vi "girpcutil_GetMethodParams.vi"(6 "timeoutMs":u32=5000, 8 "Fehler (Eingang, kein Fehler)":errorcluster, 10 "methodName":string, 11 "girpcutil_params":T1) -> (0 "Fehler (Ausgang)":errorcluster, 2 "param handle out":i32)   [LabVIEW 2016]
uses:
  girpcutil_params.ctl
panel:
  out "errMsg":u8[](array[numeric])
  out "errMsgLen":i32
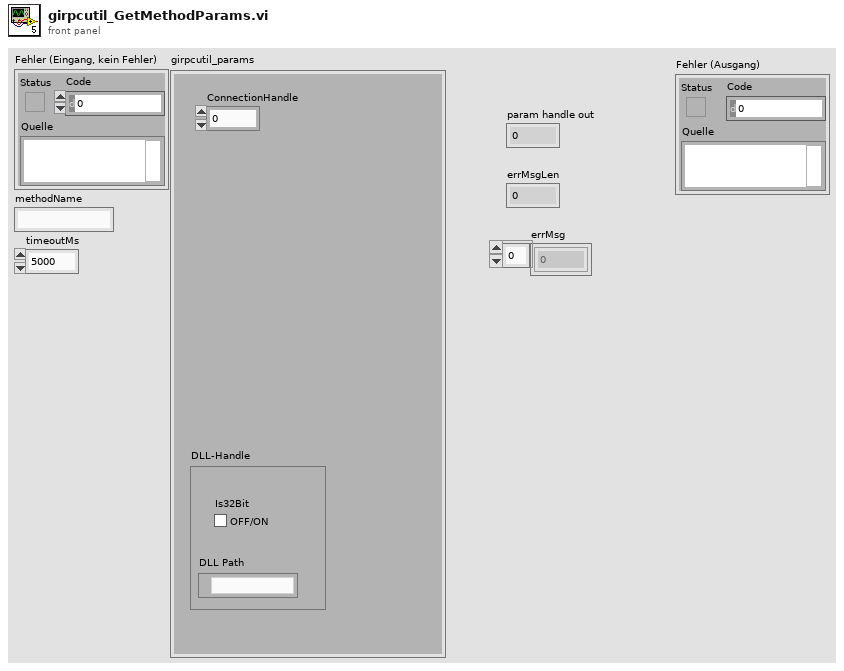
[diagram p1: front panel]
types:
  T1 = typedef "girpcutil_params.ctl" = cluster{"ConnectionHandle":i32, "DLL-Handle":cluster{"DLL Path":path, "Is32Bit":bool}}
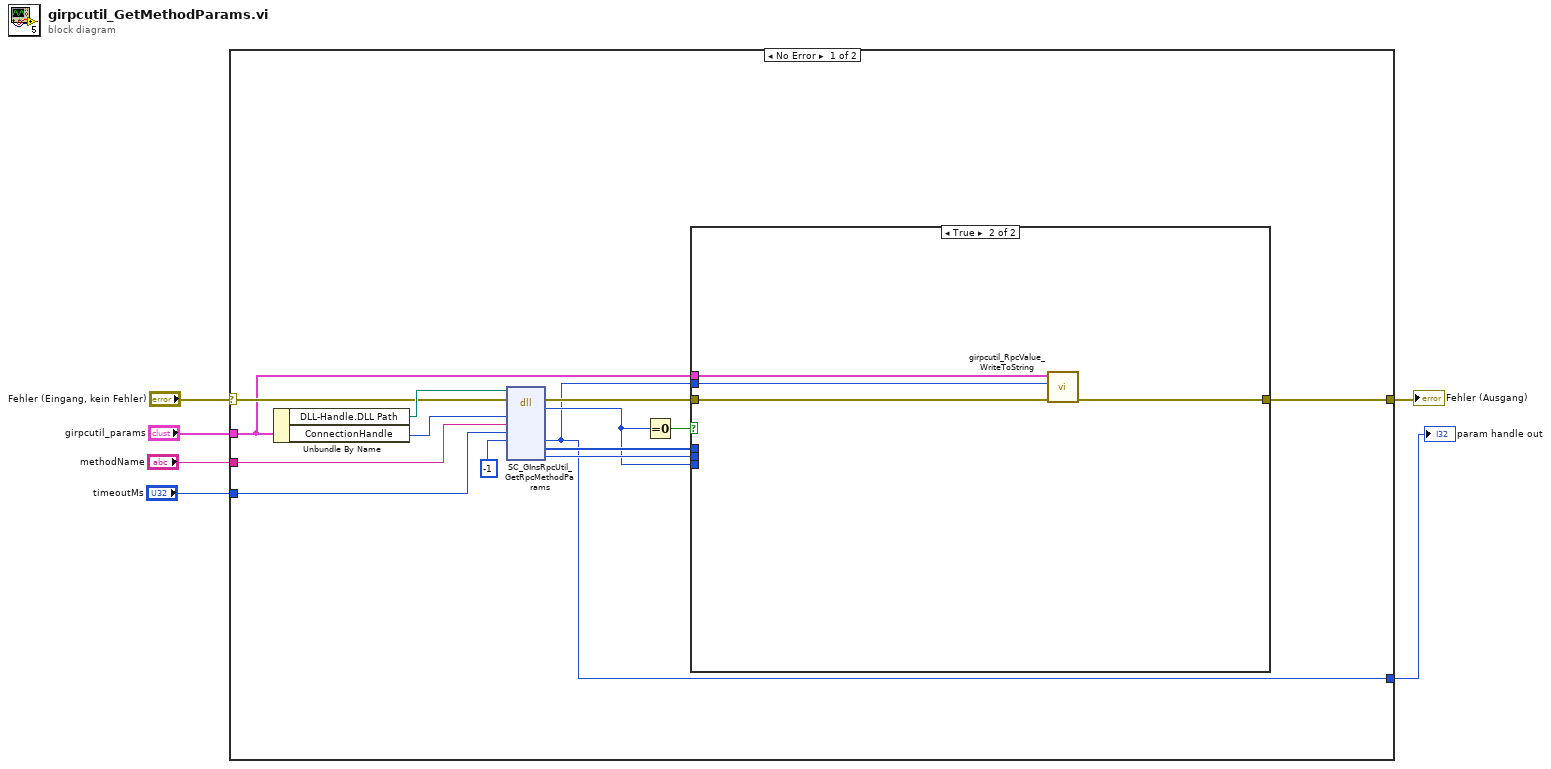
[diagram p0: block diagram]
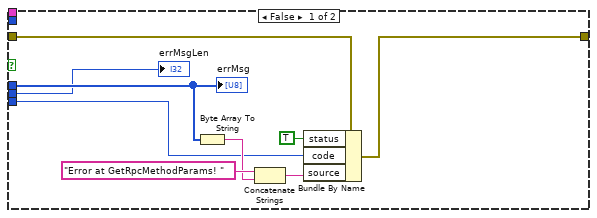
[diagram p2: hidden frame]
diagram:
  n1 = case shown="No Error" "Fehler (Eingang, kein Fehler)" {
    selector: "Fehler (Eingang, kein Fehler)" -> [w18 w34]
    tunnel: [w9 w34] -> w5
    tunnel: "girpcutil_params" -> [w7 _]
    tunnel: "methodName" -> [w16 _]
    tunnel: "timeoutMs" -> [w15 _]
    tunnel: [w8 _] -> w1
    frame No Error {
      n2 = Unbundle By Name(w7) -> ("DLL-Handle.DLL Path"=w19:path, "ConnectionHandle"=w20:i32)
      n3 = dll-call lib="?" fn="SC_GInsRpcUtil_GetRpcMethodParams"(path in=w19, error in=w18, "connectionHandle"=w20, "methodName"=w16, "timeoutMs"=w15, "params"=-1) -> (error out=w13:errorcluster, "Rückgabewert"=w10:i32, "params"=w8:i32, "errMsg"=w12:u8[], "errMsgLen"=w11:i32)  [unwired: 6 in, 1 out]
      n4 = Equal To 0?(x=w10) -> (x = 0?=w14:bool)
      n5 = case shown="True" w14 {
        tunnel: w13 -> [w23 w33]
        tunnel: [w22 w32] -> w9
        tunnel: w12 -> [w27 _]
        tunnel: w11 -> [w24 _]
        tunnel: w10 -> [w21 _]
        tunnel: w8 -> [_ w31]
        tunnel: w7 -> [_ w30]
        frame False {
          n6 = Byte Array To String(unsigned byte array=w27) -> (string=w28:string)
          n7 = Concatenate Strings("Error at GetRpcMethodParams! " ("source"), w28) -> (w26:string)
          n8 = Bundle By Name(cluster=w23, "status"=TRUE, "code"=w21, "source"=w26) -> (w22:errorcluster)
          "errMsg" <- w27
          "errMsgLen" <- w24
        }
        frame True {
          n9 = call "girpcutil_RpcValue_WriteToString.vi"("Fehler (Eingang, kein Fehler)"=w33, "value"=w31, "girpcutil_params"=w30) -> ("Fehler (Ausgang)"=w32:errorcluster)  [unwired: 8 in]
        }
      }
    }
    frame Error {
    }
  }
  "Fehler (Ausgang)" <- w5
  "param handle out" <- w1
